vi "Actor Core.vi"(8 "error in":errorcluster, 11 "Camera_Controller in":refnum<class "Camera_Controller.lvclass">) -> (0 "error out":errorcluster, 3 "Actor out":refnum<class "Actor.lvclass">)   [LabVIEW 2023, in "Camera_Controller.lvlib" / "Camera_Controller.lvclass"]
doc: "(<B>Filename</B>: Actor Framework.lvlib:Actor.lvclass:Actor Core.vi)\n\nReceives messages to the actor, reacts to them, and initiates any error handling that may shut the actor down.\n\nDescendant classes may override this VI to append parallel tasks for the actor to complete while it handles messages. Overrides use the Call Parent Class Method node."
uses:
  Camera_Controller.lvclass
  C:/Program Files/National Instruments/LabVIEW 2023/vi.lib/ActorFramework/Actor/Actor.lvclass
  <vilib>/ActorFramework/Actor/Actor.lvclass
  <vilib>/ActorFramework/Message Enqueuer/Message Enqueuer.lvclass
  typedefs/BeamProfilerData.ctl
  typedefs/ImageProcessingParameters.ctl
  <vilib>/vision/Image Controls.llb/IMAQ Image.ctl
  typedefs/Image Type.ctl
  ConcreteClasses/ConcreteInstrumentClasses/CameraClasses/Inovance_LV/Inovance_Camera/Inovance_Camera.lvclass
  ConcreteClasses/ConcreteInstrumentClasses/CameraClasses/Hama_LV/HamaCam/Hamamatsu_Camera.lvclass
  <vilib>/ActorFramework/Actor/Actor.lvclass/Actor.ctl
  <vilib>/ActorFramework/Message Enqueuer/Message Enqueuer.lvclass/Message Enqueuer.ctl
  Camera_Controller.lvclass/Camera_Controller.ctl
  Interfaces/AbstractInstrumentClasses/Cameras_LV/CameraComm Messages/Frame Ready Msg/Frame Ready Msg.lvclass/Frame Ready Msg.ctl
  <vilib>/Utility/miscctls.llb/LVMinMaxIncTypeDef.ctl
  Interfaces/AbstractInstrumentClasses/Cameras_LV/CameraInterface Messages/GetFrame Msg/GetFrame Msg.lvclass/GetFrame Msg.ctl
  Interfaces/InitDeinitInterface/InitDeinit Messages/Init Msg/Init Msg.lvclass/Init Msg.ctl
  Interfaces/AbstractInstrumentClasses/Cameras_LV/CameraInterface Messages/StartCapture Msg/StartCapture Msg.lvclass/StartCapture Msg.ctl
  <vilib>/ActorFramework/Message Enqueuer/Message Priority.ctl
  Interfaces/AbstractInstrumentClasses/Cameras_LV/CameraInterface Messages/SingleAcquisition Msg/SingleAcquisition Msg.lvclass/SingleAcquisition Msg.ctl
  Interfaces/AbstractInstrumentClasses/Cameras_LV/CameraInterface Messages/SetExposure Msg/SetExposure Msg.lvclass/SetExposure Msg.ctl
  Interfaces/AbstractInstrumentClasses/Cameras_LV/CameraInterface Messages/Set Gain Msg/Set Gain Msg.lvclass/Set Gain Msg.ctl
  <vilib>/ActorFramework/Message Enqueuer/Init from Existing Queue.vi
  <vilib>/ActorFramework/Message Enqueuer/Enqueue.vi
  Interfaces/InitDeinitInterface/InitDeinit Messages/FindInstruments Msg/FindInstruments Msg.lvclass
  C:/Program Files/National Instruments/LabVIEW 2023/vi.lib/ActorFramework/Message/Message.lvclass
  <vilib>/ActorFramework/Stop Msg/Stop Msg.lvclass
  Interfaces/AbstractInstrumentClasses/Cameras_LV/CameraComm Messages/Frame Ready Msg/Frame Ready Msg.lvclass
  Interfaces/AbstractInstrumentClasses/Cameras_LV/CameraInterface Messages/GetFrame Msg/GetFrame Msg.lvclass
  Interfaces/InitDeinitInterface/InitDeinit Messages/DeInit Msg/DeInit Msg.lvclass
  Interfaces/InitDeinitInterface/InitDeinit Messages/Init Msg/Init Msg.lvclass
  Interfaces/AbstractInstrumentClasses/Cameras_LV/CameraInterface Messages/StartCapture Msg/StartCapture Msg.lvclass
  Interfaces/AbstractInstrumentClasses/Cameras_LV/CameraInterface Messages/StopCapture Msg/StopCapture Msg.lvclass
  Interfaces/AbstractInstrumentClasses/Cameras_LV/CameraInterface Messages/SingleAcquisition Msg/SingleAcquisition Msg.lvclass
  Interfaces/AbstractInstrumentClasses/Cameras_LV/CameraInterface Messages/SetExposure Msg/SetExposure Msg.lvclass
  Interfaces/AbstractInstrumentClasses/Cameras_LV/CameraInterface Messages/Set Gain Msg/Set Gain Msg.lvclass
  Interfaces/InitDeinitInterface/InitDeinit Messages/Disconnect Msg/Disconnect Msg.lvclass
  <vilib>/ActorFramework/Message Priority Queue/Priority Enqueue.vi
  Camera_Controller.lvlib
  typedefs/typedefs.lvlib
  <userlib>/_OpenG.lib/lvdata/lvdata.llb/openg_variant.lvlib
panel:
  out "Cam Enqueuer Init":bool
  out "Stopping":bool=TRUE
  out "error out Instr":errorcluster
  out "Instrument Address":string[](array[string])
  out "Orca Enqueuer":refnum<class "Message Enqueuer.lvclass">
  out "Self Enqueuer":refnum<class "Message Enqueuer.lvclass">
  out "Inovance Enqueuer":refnum<class "Message Enqueuer.lvclass">
  out "Address Var":variant
  out "Error Var":variant
  in  "Beam Profiler Kwargs":cluster{"Pixel Size":dbl}={"Pixel Size"=2.5}
  in  "Beam Profiler Data":T1
  out "Camera Enqueuer":refnum<class "Message Enqueuer.lvclass">
  out "Brand":string[](array[string])
  out "Custom ROI":i32[](array[numeric])
  in  "Tab Control":enum32{"Camera", "Options"}(tab)
  in  "Beam Profile":bool
  in  "File Path":path
  in  "File Name":string
  in  "Save":bool
  out "Image Processed":T2(plugin-control) caption="Image"
  in  "HROI Pos":u16
  in  "HROI":bool
  out "VI":refnum<vi>
  out "Image":T2(plugin-control)
  out "Capturing":bool=TRUE
  out "FPS":dbl
  in  "Camera":u16(ring)
  out "Initialized":bool=TRUE
  in  "Open Camera":bool
  in  "Gain":dbl=1.0 min=1.0 max=32.0 step=0.1
  in  "Exposure":dbl=0.01 min=0.01 max=10000.0 step=0.01
  in  "Acquire":bool
  in  "Live":bool
  out "ROI Graph":cluster{"x0":sgl, "dx":sgl, "Pixels Line":sgl[]}(graph)={"x0"=0.0, "dx"=1.0, "Pixels Line"=[1.0, 0.0, 0.0, 0.0, 0.0, 0.0, 0.0, 0.0, 0.0, 0.0, 0.0, 0.0, 0.0, 0.0, 0.0, 0.0, 0.0, 0.0, 0.0, 0.0, 0.0, 0.0, 0.0, 0.0, 0.0, 0.0, 0.0, 0.0, 0.0, 0.0, 0.0, 0.0, 0.0, 0.0, 0.0, 0.0, 0.0, 0.0, 0.0, 0.0, 0.0, 0.0, 0.0, 0.0, 0.0, 0.0, 0.0, 0.0, 0.0, 0.0, 0.0, 0.0, 0.0, 0.0, 0.0, 0.0, 0.0, 0.0, 0.0, 0.0, 0.0, 0.0, 0.0, 0.0, 0.0, 0.0, 0.0, 0.0, 0.0, 0.0, 0.0, 0.0, 0.0, 0.0, 0.0, 0.0, 0.0, 0.0, 0.0, 0.0, 0.0, 0.0, 0.0, 0.0, 0.0, 0.0, 0.0, 0.0, 0.0, 0.0, 0.0, 0.0, 0.0, 0.0, 0.0, 0.0, 0.0, 0.0, 0.0, 0.0, 0.0, 0.0, 0.0, 0.0, 0.0, 0.0, 0.0, 0.0, 0.0, 0.0, 0.0, 0.0, 0.0, 0.0, 0.0, 0.0, 0.0, 0.0, 0.0, 0.0, 0.0, 0.0, 0.0, 0.0, 0.0, 0.0, 0.0, 0.0, 0.0, 0.0, 0.0, 0.0, 0.0, 0.0, 0.0, 0.0, 0.0, 0.0, 0.0, 0.0, 0.0, 0.0, 0.0, 0.0, 0.0, 0.0, 0.0, 0.0, 0.0, 0.0, 0.0, 0.0, 0.0, 0.0, 0.0, 0.0, 0.0, 0.0, 0.0, 0.0, 0.0, 0.0, 0.0, 0.0, 0.0, 0.0, 0.0, 0.0, 0.0, 0.0, 0.0, 0.0, 0.0, 0.0, 0.0, 0.0, 0.0, 0.0, 0.0, 0.0, 0.0, 0.0, 0.0, 0.0, 0.0, 0.0, 0.0, 0.0, 0.0, 0.0, 0.0, 0.0, 0.0, 0.0, 0.0, 0.0, 0.0, 0.0, 0.0, 0.0, 0.0, 0.0, 0.0, 0.0, 0.0, 0.0, 0.0, 0.0, 0.0, 0.0, 0.0, 0.0, 0.0, 0.0, 0.0, 0.0, 0.0, 0.0, 0.0, 0.0, 0.0, 0.0, 0.0, 0.0, 0.0, 0.0, 0.0, 0.0, 0.0, 0.0, 0.0, 0.0, 0.0, 0.0, 0.0, 0.0, 0.0, 0.0, 0.0, 0.0, 0.0, 0.0, 0.0, 0.0, 0.0, 0.0, 0.0, 0.0, 0.0, 0.0, 0.0, 0.0, 0.0, 0.0, 0.0, 0.0]}
  in  "Mode":enum16{"ROI", "Image"}(ring)
  out "ROI Parameters":cluster{"Count":sgl, "Size(um)":sgl} {"Size(um)" min=0 max=255 step=0.1 format="%.2f"; "Count" min=0 max=255 step=0.1 format="%.2f"}
  in  "Refresh Button":bool
  in  "Stop":bool
  in  "Auto?":bool
  in  "Log?":bool
  in  "Manual":cluster{sgl, sgl}(slide)={100.0, 255.0} caption="Threshold Range" scale=0.0..65535.0
  out "Beam Profile":T1
  out "Image Preview":T2(plugin-control) caption="Image"
  out "Calibration Axes":u8[][](graph)
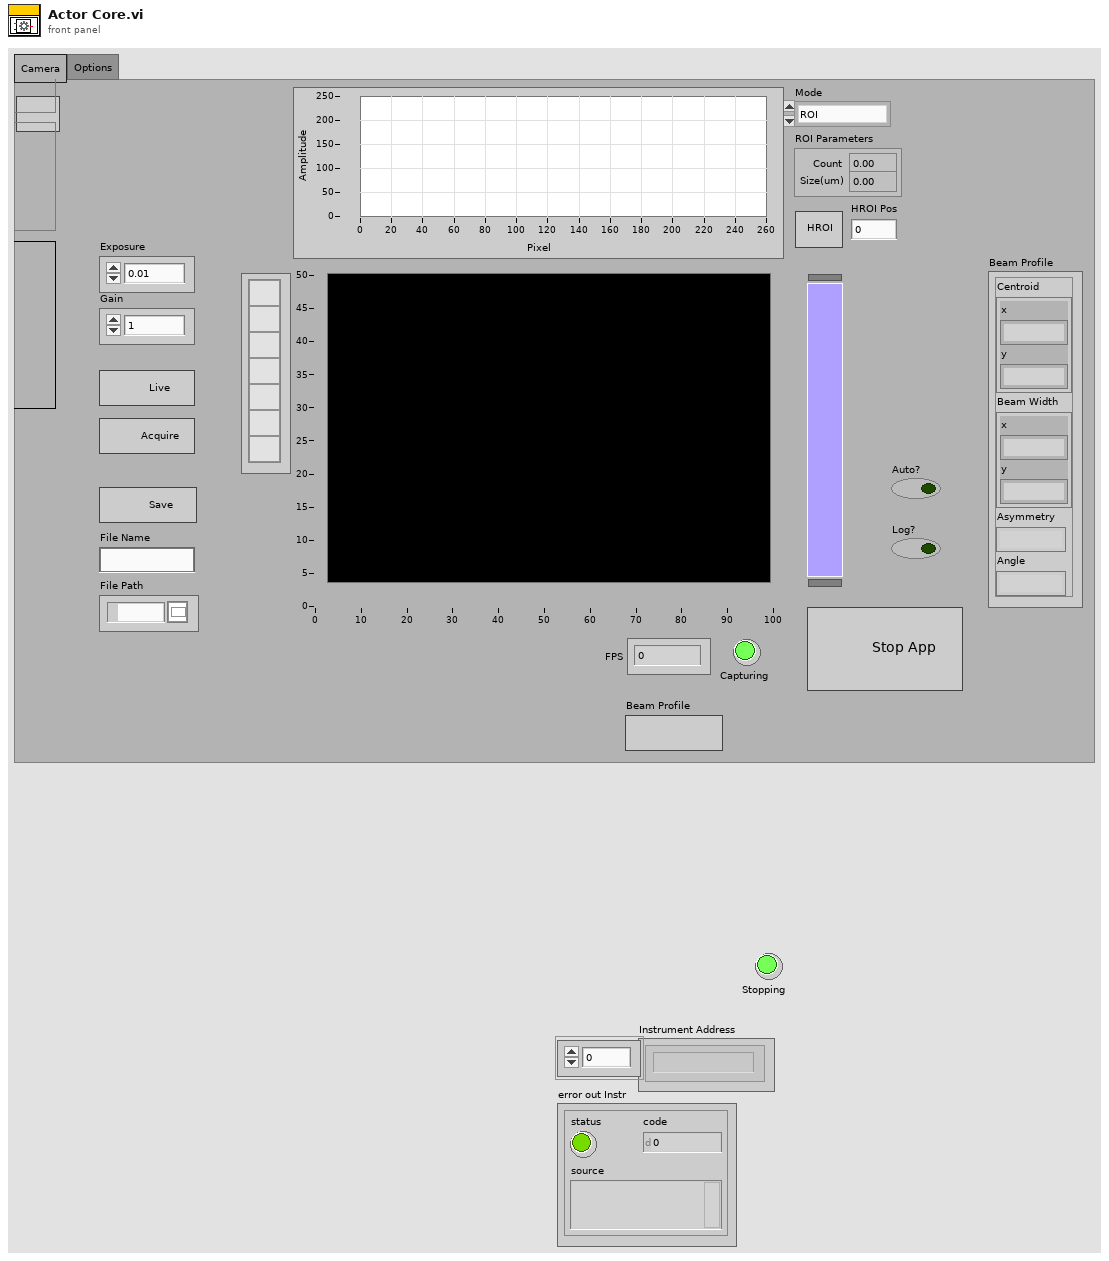
[diagram p1: front panel]
types:
  T1 = typedef "BeamProfilerData.ctl" = cluster{"Centroid":cluster{"x":string, "y":string}, "Beam Width":cluster{"x":string, "y":string}, "Asymmetry":string, "Angle":string}
  T2 = typedef "IMAQ Image.ctl" = refnum<image>
  T3 = typedef "typedefs.lvlib/ImageProcessingParameters.ctl" = cluster{"Mode":enum16{"ROI", "Image"}, "Manual LUT":cluster{"Minimum":dbl, "Maximum":dbl}, "ImageProcessed":T2, "Image ":T2, "Log?":bool, "Auto?":bool, "ROI":cluster{"Global Rectangle":i32[], "Contours":cluster{"Contour Type":u32, "ROI Type":u32, "Points":i32[]}[]}, "ROI Parameters":cluster{"Count":sgl, "Size(um)":sgl}, "Image X":i32, "Image Y":i32, "Horizontal ROI":cluster{"Global Rectangle":i32[], "Contours":cluster{"Contour Type":u32, "ROI Type":u32, "Points":i32[]}[]}, "HROI Pos":u16, "Custom ROI":cluster{"Global Rectangle":i32[], "Contours":cluster{"Contour Type":u32, "ROI Type":u32, "Points":i32[]}[]}, "Intensity Graph":u8[][], "Image Type":T4, "ImagePreview":T2}
  T4 = typedef "typedefs.lvlib/Image Type.ctl" = u32
  T5 = enum8{"Enabled", "Disabled", "Disabled and Grayed Out"}
  T6 = typedef "LVMinMaxIncTypeDef.ctl" = cluster{"Maximum":dbl, "Minimum":dbl, "Increment":dbl}
  T7 = cluster{"Global Rectangle":i32[], "Contours":cluster{"Contour Type":u32, "ROI Type":u32, "Points":i32[]}[]}
  T8 = typedef "Image Type" = u32
  T9 = typedef "Actor Framework.lvlib/Message Enqueuer.lvclass/Message Priority.ctl" = enum16{"Low", "Normal", "High"}
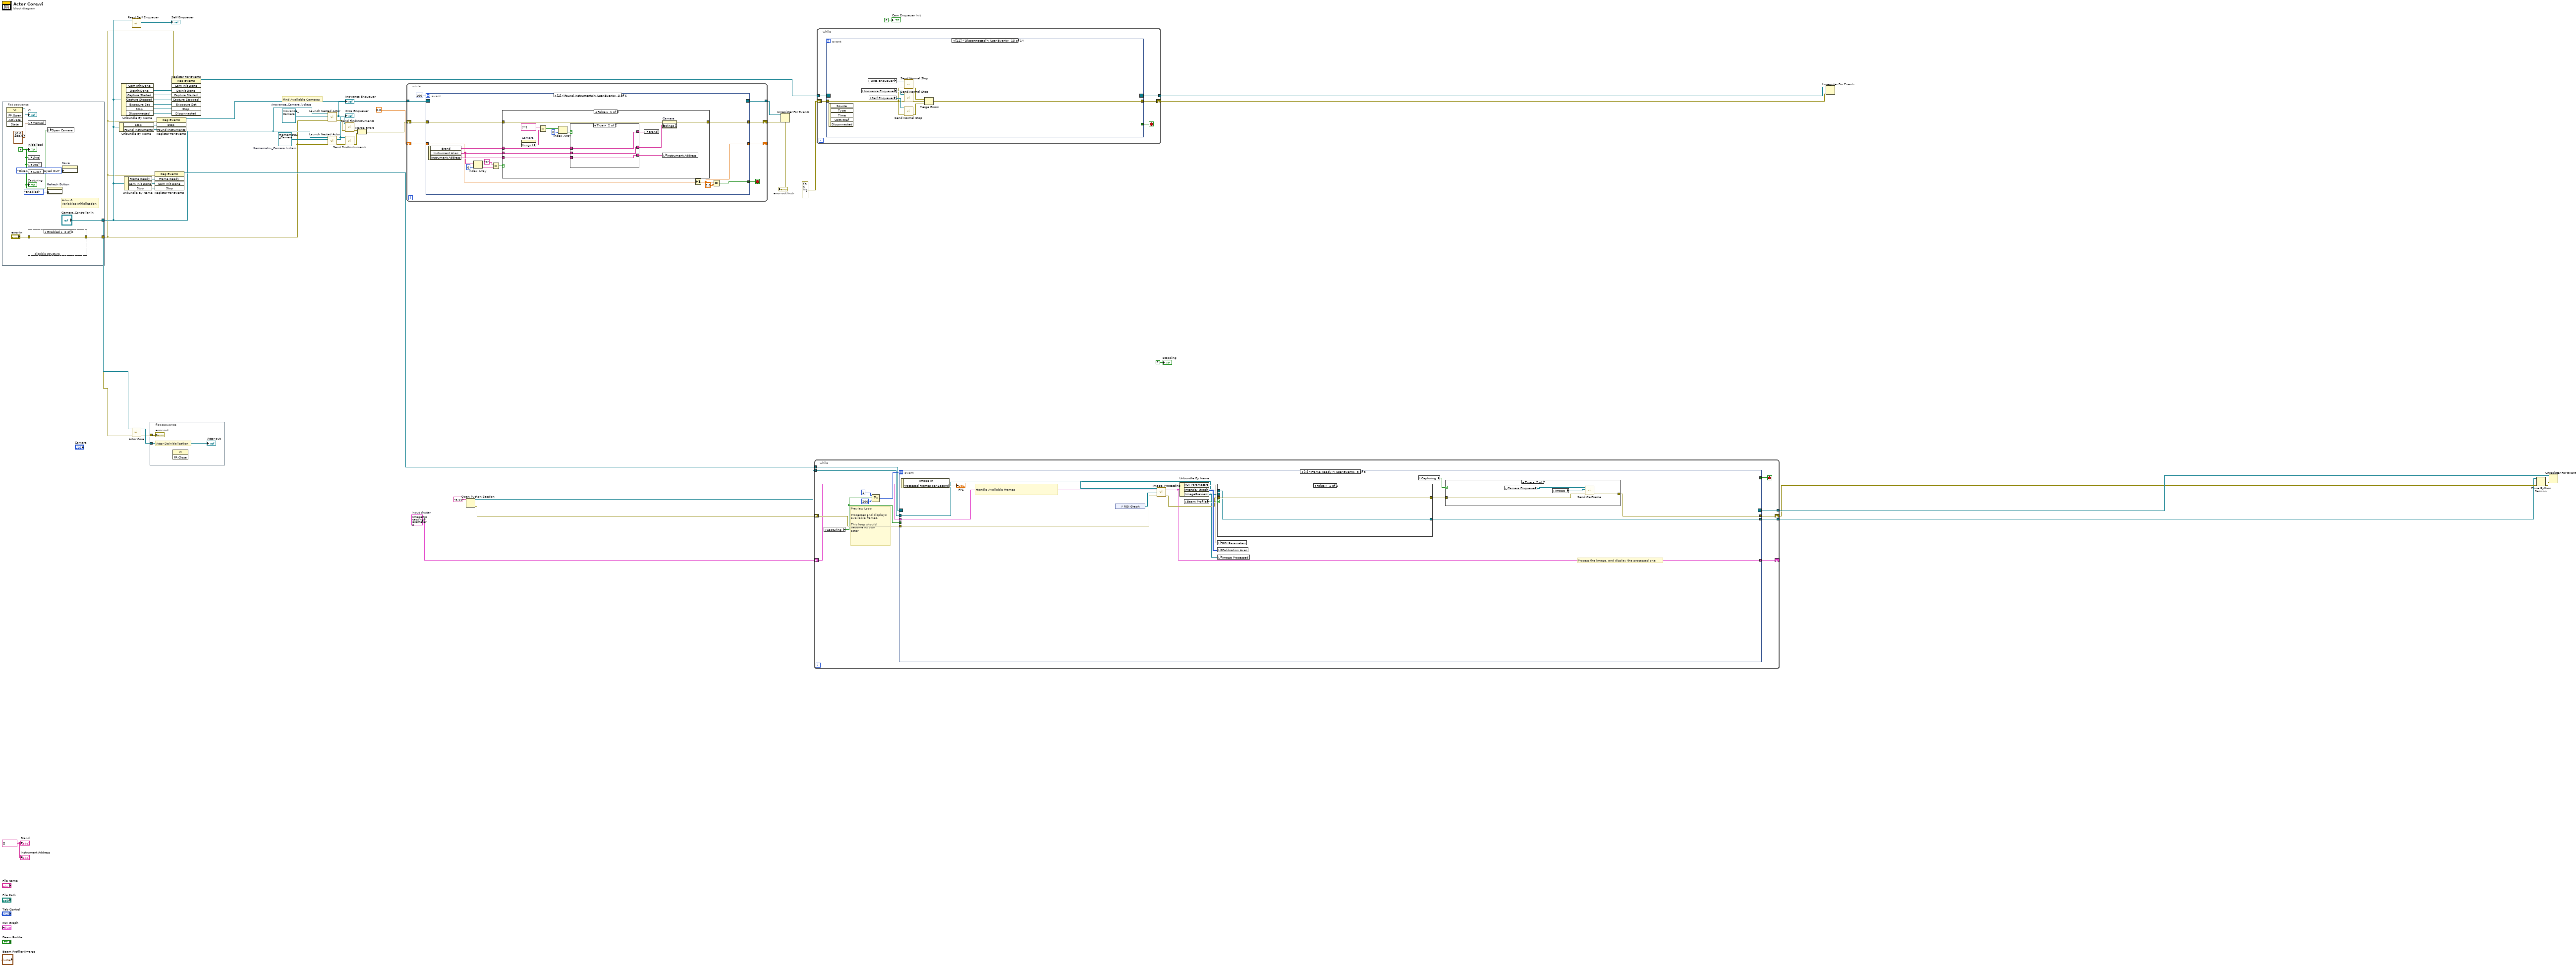
[diagram p0: block diagram]
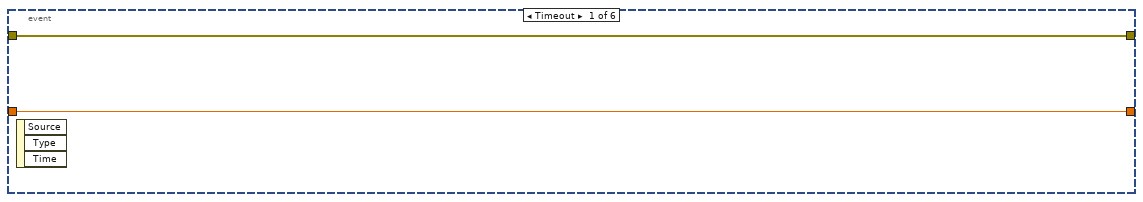
[diagram p2: hidden frame]
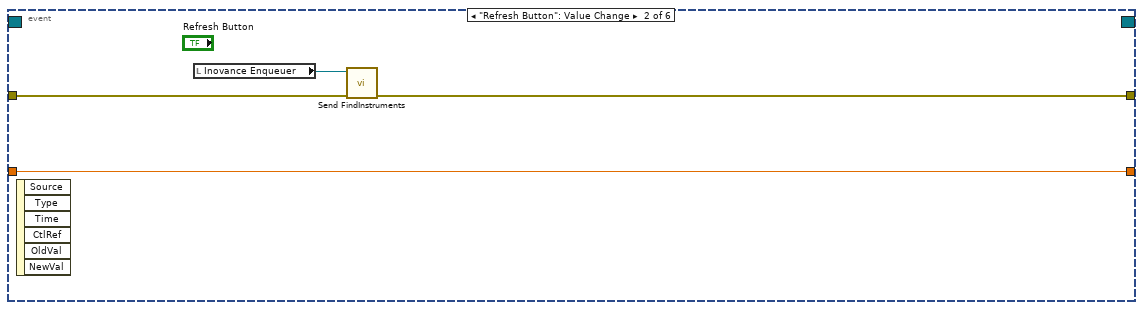
[diagram p3: hidden frame]
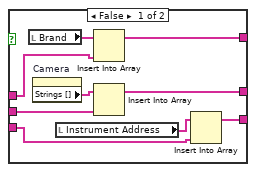
[diagram p4: hidden frame]
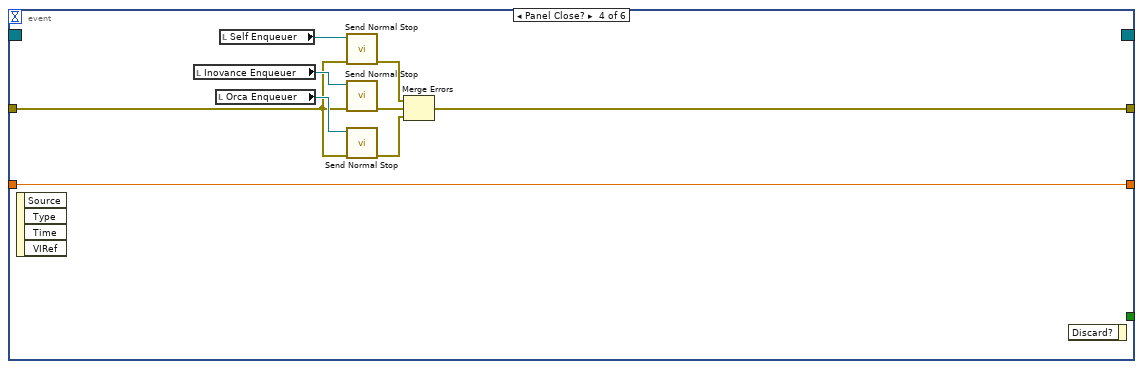
[diagram p6: hidden frame]
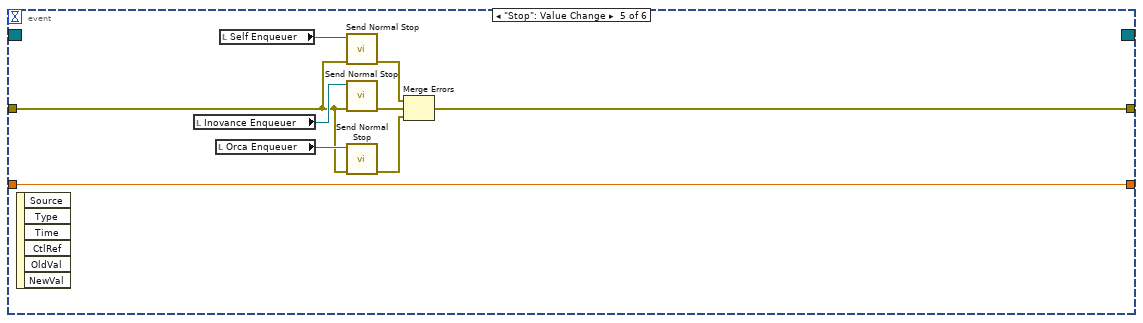
[diagram p7: hidden frame]
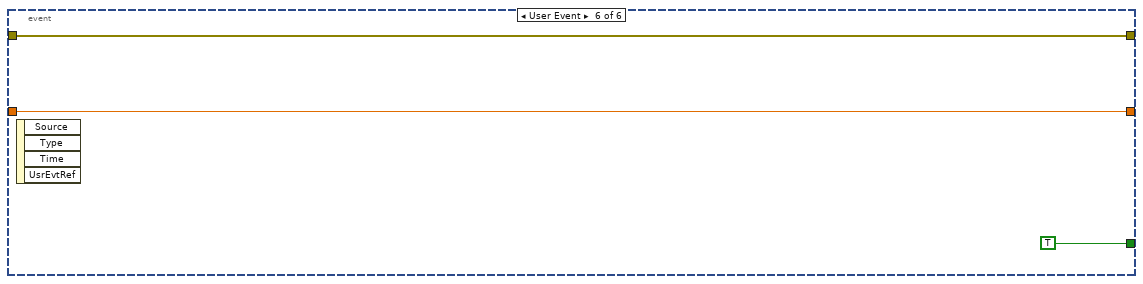
[diagram p8: hidden frame]
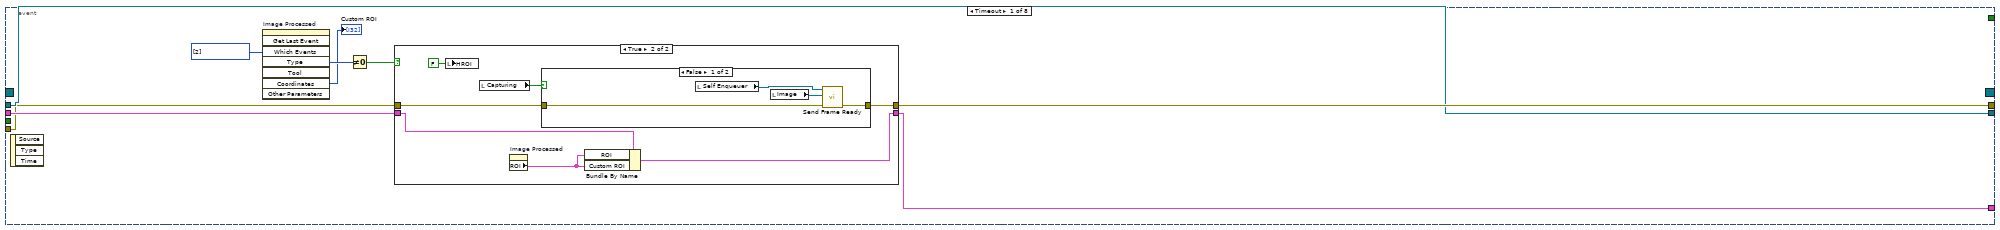
[diagram p9: hidden frame]
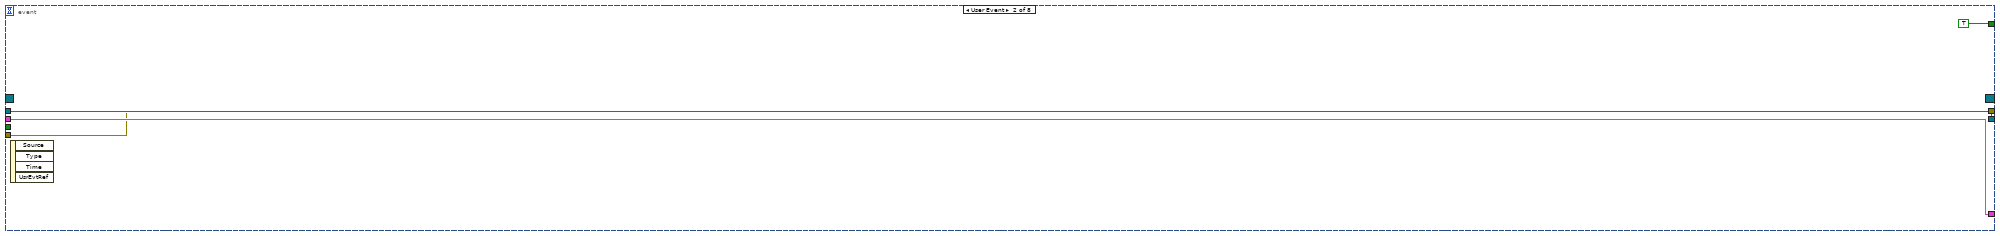
[diagram p12: hidden frame]
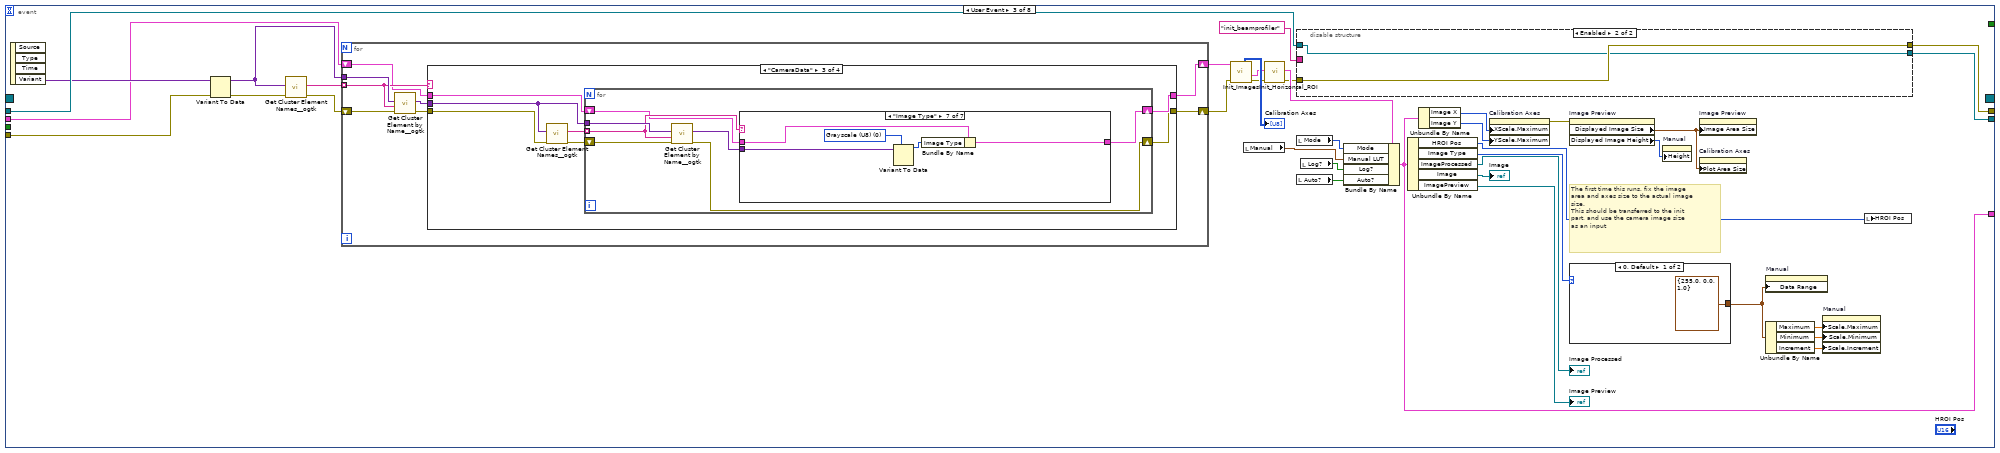
[diagram p13: hidden frame]
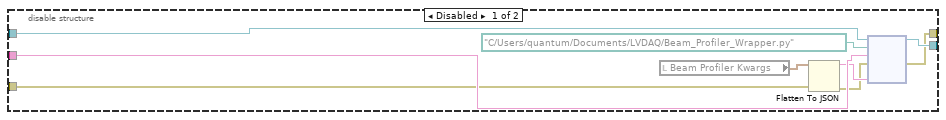
[diagram p14: hidden frame]
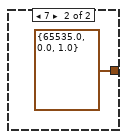
[diagram p15: hidden frame]
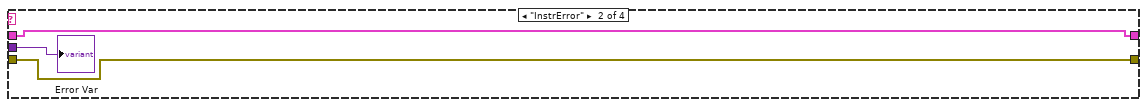
[diagram p17: hidden frame]
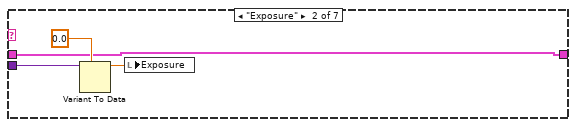
[diagram p19: hidden frame]
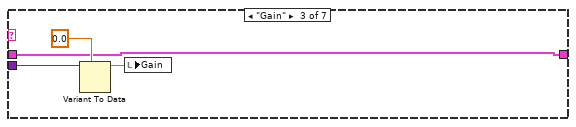
[diagram p20: hidden frame]
diagram:
  w13 = refnum<class "Hamamatsu_Camera.lvclass"> refnum  # Hamamatsu_Camera.lvclass
  w14 = refnum<class "Inovance_Camera.lvclass"> refnum  # :Inovance_Camera.lvclass
  w19 = string[] [] ("Brand")
  w37 = T3 {"Mode"=enum."Image", "Manual LUT"={"Minimum"=0.0, "Maximum"=0.0}, "ImageProcessed"=refnum, "Image "=refnum, "Log?"=FALSE, "Auto?"=FALSE, "ROI"={"Global Rectangle"=[], "Contours"=[]}, "ROI Parameters"={"Count"=0.0, "Size(um)"=0.0}, "Image X"=0, "Image Y"=0, "Horizontal ROI"={"Global Rectangle"=[], "Contours"=[]}, "HROI Pos"=0, "Custom ROI"={"Global Rectangle"=[], "Contours"=[]}, "Intensity Graph"=[], "Image Type"=7, "ImagePreview"=refnum}  # input cluster
  # "Find Available Cameras"
  n1 = flat-sequence {
    tunnel: ["Camera_Controller in"] -> w22
    tunnel: [w49] -> w2
    frame #0 {
      w53 = FALSE ("Capturing")
      # "Actor & \nVariables Initialization"
      n2 = invoke class="VI" method="FP.Open"() -> (reference out=→"VI":refnum<vi>)  [unwired: 5 in, 4 out]
      n3 = local write "Manual"(cluster{sgl, sgl} {0.0, 255.0} ("Manual")) -> ()
      n4 = local write "Live"(w53) -> ()
      n5 = local write "Log?"(w53) -> ()
      n6 = local write "Auto?"(w53) -> ()
      n7 = disable-structure shown="Enabled" {
        disable-tunnel: "error in" -> [w57 w61]
        disable-tunnel: [w56 w61] -> w49
        frame Disabled {
          n8 = Initialize Array("" ("element"), 0 ("dimension size")) -> (w60:string[])
          n9 = property on="Camera" class="Ring (strict)"(error in=w57, "Strings []"=w60) -> (error out=w56:errorcluster)  [unwired: 1 in, 1 out]
        }
        frame Enabled {
        }
      }
      n10 = local write "Open Camera"(w53) -> ()
      n11 = property on="Refresh Button" class="Bool"("DisabledEnum"=T5."Enabled" ("Disabled")) -> ()  [unwired: 2 in, 2 out]
      n12 = property on="Save" class="Bool"("DisabledEnum"=T5."Disabled and Grayed Out" ("Disabled")) -> ()  [unwired: 2 in, 2 out]
      "Capturing" <- w53
      "Initialized" <- w53
    }
  }
  n13 = Unbundle By Name(w22) -> ("Stop"=w35:refnum<user-event>, "Found Instruments"=w27:refnum<user-event>)
  n14 = Unbundle By Name(w22) -> ("Cam Init Done"=w23:refnum<user-event>, "DeInit Done"=w44:refnum<user-event>, "Capture Started"=w43:refnum<user-event>, "Capture Stopped"=w42:refnum<user-event>, "Exposure Set"=w41:refnum<user-event>, "Stop"=w36:refnum<user-event>, "Disconnected"=w4:refnum<user-event>)
  n15 = Unbundle By Name(w22) -> ("Frame Ready"=w25:refnum<user-event>, "Cam Init Done"=w24:refnum<user-event>, "Stop"=w8:refnum<user-event>)
  n16 = call <vilib>:"Read Self Enqueuer.vi"("Actor"=w22) -> ("Self Enqueuer"=→"Self Enqueuer":refnum<class "Message Enqueuer.lvclass">)  [unwired: 10 in]
  n17 = call-parent "Actor Core.vi"("error in"=w2, "Actor in"=w22) -> ("error out"=w46:errorcluster, "Actor out"=w47:refnum<class "Actor.lvclass">)  [unwired: 8 in]
  n18 = flat-sequence {
    tunnel: w47 -> [w63]
    tunnel: w46 -> [w62]
    frame #0 {
      # "Actor Deinitialization"
      n19 = invoke class="VI" method="FP.Close"() -> ()  [unwired: 3 in, 3 out]
      "error out" <- w62
      "Actor out" <- w63
    }
  }
  n20 = register-events(error in=w2, w25, w24, w8) -> (reference out=w34:refnum<event-registration>)  [unwired: 1 in, 1 out]
  n21 = register-events(error in=w2, w35, w27) -> (reference out=w5:refnum<event-registration>)  [unwired: 1 in, 1 out]
  n22 = register-events(error in=w2, w23, w44, w43, w42, w41, w36, w4) -> (reference out=w45:refnum<event-registration>)  [unwired: 1 in, 1 out]
  n23 = call <vilib>:"Launch Nested Actor.vi"("error in (no error)"=w2, "Nested Actor"=w14, "Caller Actor in"=w22) -> ("error out"=w16:errorcluster, "Nested Actor's Enqueuer"=w15:refnum<class "Message Enqueuer.lvclass">)  [unwired: 6 in, 1 out]
  "Inovance Enqueuer" <- w15
  n24 = call <vilib>:"Launch Nested Actor.vi"("error in (no error)"=w2, "Nested Actor"=w13, "Caller Actor in"=w22) -> ("error out"=w9:errorcluster, "Nested Actor's Enqueuer"=w12:refnum<class "Message Enqueuer.lvclass">)  [unwired: 6 in, 1 out]
  "Orca Enqueuer" <- w12
  n25 = call "Send FindInstruments.vi"("error in (no error)"=w16, "Message Enqueuer"=w15) -> ("error out"=w10:errorcluster)  [unwired: 8 in, 1 out]
  n26 = call "Send FindInstruments.vi"("error in (no error)"=w9, "Message Enqueuer"=w12) -> ("error out"=w11:errorcluster)  [unwired: 8 in, 1 out]
  n27 = Merge Errors(w10, w11) -> (w21:errorcluster)
  n28 = while {
    shift-right: [w71] -> w17
    shift-left: w21 -> [w70]
    tunnel: w5 -> [w68]
    shift-right: [w65] -> _
    shift-left: 0.0 -> [w66]
    tunnel: [w64] -> w18
    stop <- w69 stop-if-true
    n29 = event shown="[2] <Found Instruments>: User Event" {
      selector: w68 -> [_ _ _ _ _ _]
      dyn-events: [_ _ _ _ _ _] -> w64
      timeout: 100 -> [_ _ _ _ _ _]
      tunnel: [_ _ w89 _ _ TRUE] -> w69
      tunnel: [w73 w76 w82 w121 w130 w136] -> w71
      tunnel: w70 -> [w73 w77 w83 w118 w126 w136]
      tunnel: w66 -> [w72 w74 w79 w120 w129 w135]
      tunnel: [w72 w74 w78 w120 w129 w135] -> w65
      event Timeout {
        n30 = event-data() -> ()  [unwired: 1 in, 3 out]
      }
      event "Refresh Button": Value Change {
        n31 = event-data() -> ()  [unwired: 1 in, 6 out]
        n32 = local read "Inovance Enqueuer"() -> (w75:refnum<class "Message Enqueuer.lvclass">)
        n33 = call "Send FindInstruments.vi"("error in (no error)"=w77, "Message Enqueuer"=w75) -> ("error out"=w76:errorcluster)  [unwired: 8 in, 1 out]
      }
      event User Event {
        n34 = event-data() -> ("Brand"=w87:string[], "Instrument Alias"=w80:string[], "Instrument Address"=w81:string[])  [unwired: 1 in]
        n35 = Index Array(array=w80, index=0) -> (element=w85:string)
        n36 = Equal?(x="0", y=w85) -> (x = y?=w86:bool)
        n37 = case shown="False" w86 {
          tunnel: w80 -> [w103 _]
          tunnel: w81 -> [w102 _]
          tunnel: w87 -> [w101 _]
          tunnel: w83 -> [w98 w116]
          tunnel: [w96 w116] -> w82
          frame False {
            n38 = property on="Camera" class="Ring (strict)"() -> ("Strings []"=w93:string[])  [unwired: 2 in, 2 out]
            n39 = Equal?(x=string[] [""] ("Strings []"), y=w93) -> (x = y?=w91:bool[])
            n40 = Index Array(array=w91, index=0) -> (element=w94:bool)
            n41 = case shown="True" w94 {
              tunnel: w103 -> [w111 w115]
              tunnel: [w110 w115] -> w97
              tunnel: w101 -> [w109 w113]
              tunnel: [w106 w114] -> w99
              tunnel: [w105 w113] -> w100
              tunnel: w102 -> [w104 w114]
              frame False {
                n42 = local read "Brand"() -> (w107:string[])
                n43 = property on="Camera" class="Ring (strict)"() -> ("Strings []"=w112:string[])  [unwired: 2 in, 2 out]
                n44 = local read "Instrument Address"() -> (w108:string[])
                n45 = Insert Into Array(array=w107, new element=w109) -> (w105:string[])  [unwired: 1 in]
                n46 = Insert Into Array(array=w112, new element=w111) -> (w110:string[])  [unwired: 1 in]
                n47 = Insert Into Array(array=w108, new element=w104) -> (w106:string[])  [unwired: 1 in]
              }
              frame True {
              }
            }
            n48 = local write "Brand"(w100) -> ()
            n49 = property on="Camera" class="Ring (strict)"(error in=w98, "Strings []"=w97) -> (error out=w96:errorcluster)  [unwired: 1 in, 1 out]
            n50 = local write "Instrument Address"(w99) -> ()
          }
          frame True {
          }
        }
        n51 = Increment(x=w79) -> (x+1=w78:dbl)
        n52 = Equal?(x=w78, y=2.0) -> (x = y?=w89:bool)
      }
      event Panel Close? {
        n53 = event-data() -> ()  [unwired: 1 in, 4 out]
        n54 = local read "Inovance Enqueuer"() -> (w124:refnum<class "Message Enqueuer.lvclass">)
        n55 = local read "Orca Enqueuer"() -> (w119:refnum<class "Message Enqueuer.lvclass">)
        n56 = local read "Self Enqueuer"() -> (w125:refnum<class "Message Enqueuer.lvclass">)
        n57 = call <vilib>:"Send Normal Stop.vi"("error in (no error)"=w118, "Message Enqueuer"=w125) -> ("error out"=w123:errorcluster)  [unwired: 9 in]
        n58 = call <vilib>:"Send Normal Stop.vi"("error in (no error)"=w118, "Message Enqueuer"=w124) -> ("error out"=w122:errorcluster)  [unwired: 9 in]
        n59 = call <vilib>:"Send Normal Stop.vi"("error in (no error)"=w118, "Message Enqueuer"=w119) -> ("error out"=w117:errorcluster)  [unwired: 9 in]
        n60 = Merge Errors(w123, w122, w117) -> (w121:errorcluster)
        n61 = event-data() -> ()  [unwired: 2 in, 1 out]
      }
      event "Stop": Value Change {
        n62 = event-data() -> ()  [unwired: 1 in, 6 out]
        n63 = local read "Inovance Enqueuer"() -> (w133:refnum<class "Message Enqueuer.lvclass">)
        n64 = local read "Orca Enqueuer"() -> (w128:refnum<class "Message Enqueuer.lvclass">)
        n65 = local read "Self Enqueuer"() -> (w134:refnum<class "Message Enqueuer.lvclass">)
        n66 = call <vilib>:"Send Normal Stop.vi"("error in (no error)"=w126, "Message Enqueuer"=w134) -> ("error out"=w132:errorcluster)  [unwired: 9 in]
        n67 = call <vilib>:"Send Normal Stop.vi"("error in (no error)"=w126, "Message Enqueuer"=w133) -> ("error out"=w131:errorcluster)  [unwired: 9 in]
        n68 = call <vilib>:"Send Normal Stop.vi"("error in (no error)"=w126, "Message Enqueuer"=w128) -> ("error out"=w127:errorcluster)  [unwired: 9 in]
        n69 = Merge Errors(w132, w131, w127) -> (w130:errorcluster)
      }
      event User Event {
        n70 = event-data() -> ()  [unwired: 1 in, 4 out]
      }
    }
  }
  n71 = Open Python Session(python version="3.11" ("Python version")) -> (session out=w33:refnum<k35>, error out=w31:errorcluster)  [unwired: 2 in]
  n72 = Unregister For Events(event registration refnum=w18, error in=w17) -> (error out=→"error out Instr":errorcluster)
  n73 = while {
    tunnel: w34 -> [w150]
    tunnel: [w149] -> w40
    shift-right: [w139] -> w30
    shift-left: w31 -> [w148]
    shift-right: [w140] -> _
    shift-left: w37 -> [w143]
    tunnel: w33 -> [w142]
    tunnel: [w141] -> w28
    stop <- w138 stop-if-true
    # "Preview Loop\n\nProcesses and displays\navailable frames.\n\nThis loop should\nbecome its own\nactor"
    n74 = local read "Capturing"() -> (w144:bool)
    n75 = Select(t=1, s=w144, f=200) -> (s? t:f=w145:i32)
    n76 = event shown="[4] <Frame Ready>: User Event" {
      selector: w150 -> [_ _ _ _ _ _ _ _]
      dyn-events: [_ _ _ _ _ _ _ _] -> w149
      timeout: w145 -> [_ _ _ _ _ _ _ _]
      tunnel: [w155 w174 w212 w290 w296 w336 w360 w370] -> w139
      tunnel: w148 -> [w151 w174 w209 w292 w309 w337 w361 w371]
      tunnel: w144 -> [_ _ _ _ _ _ _ _]
      tunnel: w143 -> [w157 w176 w206 w288 w306 w338 w359 w373]
      tunnel: [w152 w176 w188 w288 w298 w331 w354 w368] -> w140
      tunnel: w142 -> [w153 w177 w214 w289 w301 w332 w355 w369]
      tunnel: [w153 w177 w213 w289 w300 w332 w355 w369] -> w141
      tunnel: [_ TRUE _ _ _ _ _ _] -> w138
      event Timeout {
        w158 = i32[] [2] items=["No Event"=0, "Click Event"=1, "Draw Event"=2, "Size Event"=4, "Scroll Event"=5, "Double Click Event"=8] ("Which Events")
        n77 = event-data() -> ()  [unwired: 1 in, 3 out]
        n78 = invoke on="Image Processed" class="ImageControl" method="Get Last Event"("Which Events"=w158) -> ("Type"=w159:i32, "Coordinates"=→"Custom ROI":i32[])  [unwired: 7 in, 6 out]
        n79 = Not Equal To 0?(x=w159) -> (x != 0?=w156:bool)
        n80 = case shown="True" w156 {
          tunnel: w157 -> [w161 w168]
          tunnel: [w161 w167] -> w152
          tunnel: w151 -> [w160 w165]
          tunnel: [w160 w164] -> w155
          frame False {
          }
          frame True {
            n81 = local write "HROI"(FALSE ("HROI")) -> ()
            n82 = local read "Capturing"() -> (w166:bool)
            n83 = property on="Image Processed" class="ImageControl"() -> ("ROI"=w163:T7)  [unwired: 2 in, 2 out]
            n84 = case shown="False" w166 {
              tunnel: w165 -> [w172 w173]
              tunnel: [w171 w173] -> w164
              frame False {
                n85 = local read "Self Enqueuer"() -> (w169:refnum<class "Message Enqueuer.lvclass">)
                n86 = local read "Image"() -> (w170:T2)
                n87 = call "Send Frame Ready.vi"("error in (no error)"=w172, "Image In"=w170, "Message Enqueuer"=w169) -> ("error out"=w171:errorcluster)  [unwired: 7 in, 1 out]
              }
              frame True {
              }
            }
            n88 = Bundle By Name(cluster=w168, "ROI"=w163, "Custom ROI"=w163) -> (w167:T3)
          }
        }
      }
      event User Event {
        n89 = event-data() -> ()  [unwired: 1 in, 4 out]
      }
      event User Event {
        # "The first time this runs, fix the image\narea and axes size to the actual image\nsize.\nThis should be transferred to the init\npart, and use the camera image size\nas an input"
        n90 = event-data() -> ("Variant"=w210:variant)  [unwired: 1 in, 3 out]
        n91 = Variant To Data(error in=w209, Variant=w210) -> (data=w207:variant, error out=w195:errorcluster)  [unwired: 1 in]
        n92 = call <userlib>:"Get Cluster Element Names__ogtk.vi"("error in (no error)"=w195, "Cluster"=w207) -> ("error out"=w196:errorcluster, "Element Names"=w208:string[])  [unwired: 8 in]
        n93 = for {
          tunnel: w208 -> [w234] mode=indexing
          tunnel: w207 -> [w235]
          shift-right: [w229] -> w194
          shift-left: w196 -> [w230]
          shift-right: [w228] -> w205
          shift-left: w206 -> [w232]
          n94 = call <userlib>:"Get Cluster Element by Name__ogtk.vi"("error in (no error)"=w230, "Element Name"=w234, "Cluster"=w235) -> ("error out"=w231:errorcluster, "VElement"=w233:variant)  [unwired: 6 in, 1 out]
          n95 = case shown="\"CameraData\"" w234 {
            tunnel: w233 -> [_ w240 w246 w287]
            tunnel: w232 -> [w237 w239 w245 w286]
            tunnel: [w237 w239 w244 w286] -> w228
            tunnel: w231 -> [w236 w238 w243 w285]
            tunnel: [w236 w238 w241 w285] -> w229
            frame "False", Default {
            }
            frame "InstrError" {
              "Error Var" <- w240
            }
            frame "CameraData" {
              n96 = call <userlib>:"Get Cluster Element Names__ogtk.vi"("error in (no error)"=w243, "Cluster"=w246) -> ("error out"=w242:errorcluster, "Element Names"=w247:string[])  [unwired: 8 in]
              n97 = for {
                tunnel: w247 -> [w253] mode=indexing
                tunnel: w246 -> [w254]
                shift-right: [w248] -> w241
                shift-left: w242 -> [w249]
                shift-right: [w250] -> w244
                shift-left: w245 -> [w251]
                n98 = call <userlib>:"Get Cluster Element by Name__ogtk.vi"("error in (no error)"=w249, "Element Name"=w253, "Cluster"=w254) -> ("error out"=w248:errorcluster, "VElement"=w252:variant)  [unwired: 6 in, 1 out]
                n99 = case shown="\"Image Type\"" w253 {
                  tunnel: w252 -> [_ w259 w263 w268 w273 w279 w284]
                  tunnel: w251 -> [w255 w256 w260 w266 w270 w274 w283]
                  tunnel: [w255 w256 w260 w265 w269 w274 w282] -> w250
                  frame "False", Default {
                  }
                  frame "Exposure" {
                    n100 = Variant To Data(type=0.0, Variant=w259) -> (data=w257:dbl)  [unwired: 1 in, 1 out]
                    n101 = local write "Exposure"(w257) -> ()
                  }
                  frame "Gain" {
                    n102 = Variant To Data(type=0.0, Variant=w263) -> (data=w261:dbl)  [unwired: 1 in, 1 out]
                    n103 = local write "Gain"(w261) -> ()
                  }
                  frame "Image XDim" {
                    n104 = Variant To Data(type=u16 0 ("Image XDim"), Variant=w268) -> (data=w264:u16)  [unwired: 1 in, 1 out]
                    n105 = Bundle By Name(cluster=w266, "Image X"=w264) -> (w265:T3)
                  }
                  frame "Image YDim" {
                    n106 = Variant To Data(type=u16 0 ("Image XDim"), Variant=w273) -> (data=w271:u16)  [unwired: 1 in, 1 out]
                    n107 = Bundle By Name(cluster=w270, "Image Y"=w271) -> (w269:T3)
                  }
                  frame "Pixel Size" {
                    n108 = Variant To Data(type=0.0 ("Image XDim"), Variant=w279) -> (data=w275:dbl)  [unwired: 1 in, 1 out]
                    n109 = local read "Beam Profiler Kwargs"() -> (w276:cluster{"Pixel Size":dbl})
                    n110 = Bundle By Name(cluster=w276, "Pixel Size"=w275) -> (w277:cluster{"Pixel Size":dbl})
                    n111 = local write "Beam Profiler Kwargs"(w277) -> ()
                  }
                  frame "Image Type" {
                    w280 = T8 0 items=["Grayscale (U8)", "Grayscale (I16)", "Grayscale (SGL)", "Complex (CSG)", "RGB (U32)", "HSL (U32)", "RGB (U64)", "Grayscale (U16)"] ("Image Type")
                    n112 = Variant To Data(type=w280, Variant=w284) -> (data=w281:T8)  [unwired: 1 in, 1 out]
                    n113 = Bundle By Name(cluster=w283, "Image Type"=w281) -> (w282:T3)
                  }
                }
              }
            }
            frame "Address" {
              "Address Var" <- w287
            }
          }
        }
        n114 = call "Init_Images.vi"("error in (no error)"=w194, "input cluster in"=w205) -> ("error out"=w193:errorcluster, "input cluster out"=w197:T3, "Image Pixels (U8)"=→"Calibration Axes":u8[][])  [unwired: 7 in]
        n115 = local read "Manual"() -> (w203:cluster{sgl, sgl})
        n116 = call "Init_Horizontal_ROI.vi"("error in (no error)"=w193, "input cluster"=w197) -> ("error out"=w192:errorcluster, "output cluster"=w200:T3)  [unwired: 8 in]
        n117 = disable-structure shown="Enabled" {
          disable-tunnel: w214 -> [w223 w224]
          disable-tunnel: [w222 w224] -> w213
          disable-tunnel: [w221 w225] -> w212
          disable-tunnel: "init_beamprofiler" ("function name") -> [w219 _]
          disable-tunnel: w192 -> [w216 w225]
          frame Disabled {
            n118 = local read "Beam Profiler Kwargs"() -> (w217:cluster{"Pixel Size":dbl})
            n119 = Flatten To JSON(anything=w217, error in (no error)=w216) -> (JSON string=w218:string, 11:w215:errorcluster)  [unwired: 1 in]
            n120 = node(w223, path "C:/Users/quantum/Documents/LVDAQ/Beam_Profiler_Wrapper.py" ("module path"), w219, w215, w218) -> (w222:refnum<k35>, w221:errorcluster)  [unwired: 3 in, 2 out]
          }
          frame Enabled {
          }
        }
        n121 = local read "Mode"() -> (w204:enum16{"ROI", "Image"})
        n122 = local read "Auto?"() -> (w201:bool)
        n123 = local read "Log?"() -> (w202:bool)
        n124 = Bundle By Name(cluster=w200, "Mode"=w204, "Manual LUT"=w203, "Log?"=w202, "Auto?"=w201) -> (w188:T3)
        n125 = Unbundle By Name(w188) -> ("HROI Pos"=w198:u16, "Image Type"=w191:T4, "ImageProcessed"=→"Image Processed":T2, "Image"=→"Image":T2, "ImagePreview"=→"Image Preview":T2)
        n126 = Unbundle By Name(w188) -> ("Image X"=w185:i32, "Image Y"=w184:i32)
        n127 = property on="Calibration Axes" class="IntGraph (strict)"("XScale.Maximum"=w185, "YScale.Maximum"=w184) -> (error out=w183:errorcluster)  [unwired: 2 in, 1 out]
        n128 = property on="Image Preview" class="ImageControl"(error in=w183) -> ("Displayed Image Size"=w187:cluster{"Width":u32, "Height":u32}, "Displayed Image Height"=w186:u32)  [unwired: 1 in, 2 out]
        n129 = case shown="0, Default" w191 {
          tunnel: [T6 {"Maximum"=255.0, "Minimum"=0.0, "Increment"=1.0} ("Data Entry Limits") T6 {"Maximum"=65535.0, "Minimum"=0.0, "Increment"=1.0} ("Data Entry Limits")] -> w181
          frame 0, Default {
          }
          frame 7 {
          }
        }
        n130 = property on="Manual" class="Slide (strict)"("Height"=w186) -> ()  [unwired: 2 in, 2 out]
        n131 = property on="Image Preview" class="ImageControl"("Image Area Size"=w187) -> ()  [unwired: 2 in, 2 out]
        n132 = property on="Calibration Axes" class="IntGraph (strict)"("Plot Area Size"=w187) -> ()  [unwired: 2 in, 2 out]
        n133 = property on="Manual" class="Slide (strict)"("Data Range"=w181) -> ()  [unwired: 2 in, 2 out]
        n134 = Unbundle By Name(w181) -> ("Maximum"=w178:dbl, "Minimum"=w180:dbl, "Increment"=w179:dbl)
        n135 = property on="Manual" class="Slide (strict)"("Scale.Maximum"=w178, "Scale.Minimum"=w180, "Scale.Increment"=w179) -> ()  [unwired: 2 in, 2 out]
        n136 = local write "HROI Pos"(w198) -> ()
      }
      event "Save": Value Change {
        n137 = event-data() -> ()  [unwired: 1 in, 6 out]
        n138 = Unbundle By Name(w288) -> ("ImageProcessed"=w291:T2)
        n139 = local read "File Name"() -> (w293:string)
        n140 = local read "File Path"() -> (w294:path)
        n141 = call "Save_Image.vi"("error in (no error)"=w292, "String"=w293, "Scan Save Path"=w294, "Refnum in"=w291) -> ("error out"=w290:errorcluster)  [unwired: 7 in]
      }
      event User Event {
        # "Process the image, and display the processed one"
        # "Handle Available Frames"
        n142 = event-data() -> ("Image In"=w307:T2, "Processed Frames per Second"=→"FPS":dbl)  [unwired: 1 in]
        n143 = control-ref of="ROI Graph"() -> (w308:refnum<vi>)
        n144 = call "Image_Processing.vi"("Image"=w307, "input cluster"=w306, "WaveformGraph in"=w308, "error in (no error)"=w309) -> ("output cluster"=w298:T3, "error out"=w302:errorcluster)  [unwired: 14 in]
        n145 = Unbundle By Name(w298) -> ("ROI Parameters"=w304:cluster{"Count":sgl, "Size(um)":sgl}, "Intensity Graph"=w305:u8[][], "ImagePreview"=w299:T2)
        n146 = local read "Beam Profile"() -> (w303:bool)
        n147 = case shown="False" w303 {
          tunnel: w302 -> [w317 w320]
          tunnel: [w317 w326] -> w297
          tunnel: w301 -> [w316 w330]
          tunnel: [w316 w329] -> w300
          tunnel: w299 -> [_ w321]
          frame False {
          }
          frame True {
            w325 = "calculate_values" ("function name")
            n148 = call "IMAQ ImageToArray"("error in (no error)"=w320, "Image"=w321) -> ("error out"=w318:errorcluster, "Image Pixels (U8)"=w319:u8[][])  [unwired: 2 in, 3 out]
            n149 = node(w330, path "C:/Users/quantum/Documents/LVDAQ/Beam_Profiler_Wrapper.py" ("module path"), w325, w318, w325, w319) -> (w329:refnum<k35>, w322:errorcluster, w327:string)  [unwired: 1 in, 2 out]
            n150 = Unflatten From JSON(JSON string=w327, type and defaults="Beam Profiler Data", error in (no error)=w322) -> (value=→"Beam Profile":T1, error out=w326:errorcluster)  [unwired: 4 in]
          }
        }
        n151 = local write "ROI Parameters"(w304) -> ()
        n152 = local write "Calibration Axes"(w305) -> ()
        n153 = local write "Image Processed"(w299) -> ()
        n154 = local read "Capturing"() -> (w295:bool)
        n155 = case shown="True" w295 {
          tunnel: w297 -> [w311 w313]
          tunnel: [w311 w312] -> w296
          frame False {
          }
          frame True {
            n156 = local read "Camera Enqueuer"() -> (w314:refnum<class "Message Enqueuer.lvclass">)
            n157 = local read "Image"() -> (w315:T2)
            n158 = call "Send GetFrame.vi"("error in (no error)"=w313, "Image In"=w315, "Message Enqueuer"=w314) -> ("error out"=w312:errorcluster)  [unwired: 7 in, 1 out]
          }
        }
      }
      event "Auto?", "Log?", "Manual", "Mode": Value Change {
        n159 = event-data() -> ()  [unwired: 1 in, 6 out]
        n160 = Bundle By Name(cluster=w338, "Mode"="Mode", "Manual LUT"="Manual", "Log?"="Log?", "Auto?"="Auto?") -> (w334:T3)
        n161 = control-ref of="ROI Graph"() -> (w339:refnum<vi>)
        n162 = local read "Capturing"() -> (w343:bool)
        n163 = local read "Image"() -> (w333:T2)
        n164 = case shown="False" w343 {
          tunnel: w339 -> [w351 _]
          tunnel: [w350 w353] -> w336
          tunnel: w337 -> [w349 w353]
          tunnel: w334 -> [w348 w352]
          tunnel: [w346 w352] -> w331
          tunnel: w333 -> [w347 _]
          frame False {
            n165 = call "Image_Processing.vi"("Image"=w347, "input cluster"=w348, "WaveformGraph in"=w351, "error in (no error)"=w349) -> ("output cluster"=w346:T3, "error out"=w350:errorcluster)  [unwired: 14 in]
            n166 = Unbundle By Name(w346) -> ("ImageProcessed"=w344:T2, "ROI Parameters"=→"ROI Parameters":cluster{"Count":sgl, "Size(um)":sgl})
            n167 = local write "Image Processed"(w344) -> ()
          }
          frame True {
          }
        }
      }
      event "HROI Pos": Value Change {
        n168 = event-data() -> ("NewVal"=w357:u16)  [unwired: 1 in, 5 out]
        n169 = Bundle By Name(cluster=w359, "HROI Pos"=w357) -> (w358:T3)
        n170 = local read "HROI"() -> (w356:bool)
        n171 = case shown="True" w356 {
          tunnel: w361 -> [w362 w367]
          tunnel: [w362 w366] -> w360
          tunnel: [w363 w365] -> w354
          tunnel: w358 -> [w363 w364]
          frame False {
          }
          frame True {
            n172 = call "Set_Horizontal_ROI.vi"("error in (no error)"=w367, "input cluster"=w364) -> ("error out"=w366:errorcluster, "output cluster"=w365:T3)  [unwired: 8 in]
          }
        }
      }
      event "HROI": Value Change {
        n173 = event-data() -> ("NewVal"=w372:bool)  [unwired: 1 in, 5 out]
        n174 = case shown="True" w372 {
          tunnel: w373 -> [w378 w383]
          tunnel: [w376 w382] -> w368
          tunnel: w371 -> [w375 w380]
          tunnel: [w374 w380] -> w370
          frame True {
            n175 = flat-sequence {
              tunnel: [w379] -> w377
              tunnel: w378 -> [w379]
              frame #0 {
                n176 = invoke on="Image Processed" class="ImageControl" method="Clear ROI"() -> ()  [unwired: 3 in, 3 out]
              }
            }
            n177 = call "Set_Horizontal_ROI.vi"("error in (no error)"=w375, "input cluster"=w377) -> ("error out"=w374:errorcluster, "output cluster"=w376:T3)  [unwired: 8 in]
          }
          frame False {
            n178 = Unbundle By Name(w383) -> ("Custom ROI"=w381:T7)
            n179 = Bundle By Name(cluster=w383, "ROI"=w381) -> (w382:T3)
          }
        }
      }
    }
  }
  n180 = while {
    shift-right: [w385] -> w39
    shift-left: errorcluster {"status"=FALSE, "code"=0, "source"=""} ("error out") -> [w386]
    tunnel: w45 -> [w388]
    tunnel: [w387] -> w38
    stop <- w384 stop-if-true
    n181 = event shown="[12] <Disconnected>: User Event" {
      selector: w388 -> [_ _ _ _ _ _ _ _ _ _ _ _ _ _]
      dyn-events: [_ _ _ _ _ _ _ _ _ _ _ _ _ _] -> w387
      timeout: _ -> [_ _ _ _ _ _ _ _ _ _ _ _ _ _]
      tunnel: [w390 w417 w433 w441 w450 w461 w487 w497 w503 w509 w518 w520 w526 w532] -> w385
      tunnel: w386 -> [w389 w420 w434 w442 w452 w462 w492 w497 w502 w510 w518 w521 w524 w532]
      tunnel: [_ _ _ _ _ _ _ _ _ _ _ _ _ TRUE] -> w384
      event "Open Camera": Value Change {
        n182 = event-data() -> ("NewVal"=w391:bool)  [unwired: 1 in, 5 out]
        n183 = case shown="False" w391 {
          tunnel: [w393 w397] -> w390
          tunnel: w389 -> [w394 w400]
          frame False {
            n184 = local write "Capturing"(FALSE ("Capturing")) -> ()
            n185 = local read "Camera Enqueuer"() -> (w392:refnum<class "Message Enqueuer.lvclass">)
            n186 = call "Send DeInit.vi"("error in (no error)"=w394, "Message Enqueuer"=w392) -> ("error out"=w393:errorcluster)  [unwired: 8 in, 1 out]
          }
          frame True {
            n187 = property on="Camera" class="Ring (strict)"() -> ("Value"=w407:u16)  [unwired: 2 in, 2 out]
            n188 = property on="Brand" class="Arr (strict)"() -> ("Value"=w406:string[])  [unwired: 2 in, 2 out]
            n189 = local write "Cam Enqueuer Init"(TRUE ("Initialized")) -> ()
            n190 = Index Array(array=w406, index=w407) -> (element=w405:string)
            n191 = case shown="\"INOVISION\"" w405 {
              tunnel: [refnum<class "Message Enqueuer.lvclass"> refnum ("Nested Actor's Enqueuer") w413 w416] -> w403
              tunnel: w400 -> [w408 w411 _]
              tunnel: [w408 w410 w414] -> w399
              frame "False", Default {
              }
              frame "INOVISION" {
                n192 = local read "Orca Enqueuer"() -> (w412:refnum<class "Message Enqueuer.lvclass">)
                n193 = local read "Inovance Enqueuer"() -> (w413:refnum<class "Message Enqueuer.lvclass">)
                n194 = call <vilib>:"Send Normal Stop.vi"("error in (no error)"=w411, "Message Enqueuer"=w412) -> ("error out"=w410:errorcluster)  [unwired: 9 in]
              }
              frame "Hamamatsu" {
                n195 = local read "Inovance Enqueuer"() -> (w415:refnum<class "Message Enqueuer.lvclass">)
                n196 = local read "Orca Enqueuer"() -> (w416:refnum<class "Message Enqueuer.lvclass">)
                n197 = call <vilib>:"Send Normal Stop.vi"("Message Enqueuer"=w415) -> ("error out"=w414:errorcluster)  [unwired: 10 in]
              }
            }
            "Camera Enqueuer" <- w403
            n198 = local read "Instrument Address"() -> (w402:string[])
            n199 = property on="Camera" class="Ring (strict)"() -> ("Value"=w404:u16)  [unwired: 2 in, 2 out]
            n200 = Index Array(array=w402, index=w404) -> (element=w401:string)
            n201 = call "Send Init.vi"("error in (no error)"=w400, "Address"=w401, "Message Enqueuer"=w403) -> ("error out"=w398:errorcluster)  [unwired: 7 in, 1 out]
            n202 = Merge Errors(w399, w398) -> (w397:errorcluster)
          }
        }
      }
      event "Live": Value Change {
        n203 = event-data() -> ("NewVal"=w419:bool)  [unwired: 1 in, 5 out]
        n204 = case shown="False" w419 {
          tunnel: w420 -> [w427 w431]
          tunnel: [w426 w428] -> w418
          frame True {
            n205 = local read "Camera Enqueuer"() -> (w425:refnum<class "Message Enqueuer.lvclass">)
            n206 = call "Send StartCapture.vi"("error in (no error)"=w427, "Message Enqueuer"=w425) -> ("error out"=w426:errorcluster)  [unwired: 8 in, 1 out]
          }
          frame False {
            n207 = local read "Camera Enqueuer"() -> (w429:refnum<class "Message Enqueuer.lvclass">)
            n208 = call "Send StopCapture.vi"("Message Priority (Normal)"=Message_Priority."High", "error in (no error)"=w431, "Message Enqueuer"=w429) -> ("error out"=w428:errorcluster)  [unwired: 7 in, 1 out]
          }
        }
        n209 = case shown="Error .." w418 {
          selector: w418 -> [_ w424]
          tunnel: [errorcluster {"status"=FALSE, "code"=0, "source"=""} ("error out") errorcluster {"status"=FALSE, "code"=0, "source"=""} ("error out")] -> w417
          frame No Error {
          }
          frame Error {
            n210 = Unbundle By Name(w424) -> ("source"=w423:string)
            n211 = One Button Dialog(message=w423) -> ()  [unwired: 1 in, 1 out]
          }
        }
      }
      event "Acquire": Value Change {
        n212 = event-data() -> ()  [unwired: 1 in, 6 out]
        n213 = local read "Capturing"() -> (w432:bool)
        n214 = case shown="False" w432 {
          tunnel: w434 -> [w437 w439]
          tunnel: [w436 w439] -> w433
          frame False {
            n215 = local read "Camera Enqueuer"() -> (w435:refnum<class "Message Enqueuer.lvclass">)
            n216 = local read "Image"() -> (w438:T2)
            n217 = call "Send SingleAcquisition.vi"("error in (no error)"=w437, "Image"=w438, "Message Enqueuer"=w435) -> ("error out"=w436:errorcluster)  [unwired: 7 in, 1 out]
          }
          frame True {
          }
        }
      }
      event "Exposure": Value Change {
        n218 = event-data() -> ("NewVal"=w443:dbl)  [unwired: 1 in, 5 out]
        n219 = local read "Initialized"() -> (w440:bool)
        n220 = case shown="True" w440 {
          tunnel: w443 -> [_ w449]
          tunnel: w442 -> [w444 w448]
          tunnel: [w444 w447] -> w441
          frame False {
          }
          frame True {
            n221 = local read "Camera Enqueuer"() -> (w445:refnum<class "Message Enqueuer.lvclass">)
            n222 = call "Send SetExposure.vi"("Message Priority (Normal)"=Message_Priority."High", "error in (no error)"=w448, "Exposure(ms)"=w449, "Message Enqueuer"=w445) -> ("error out"=w447:errorcluster)  [unwired: 6 in, 1 out]
          }
        }
      }
      event "Gain": Value Change {
        n223 = event-data() -> ("NewVal"=w451:dbl)  [unwired: 1 in, 5 out]
        n224 = local read "Initialized"() -> (w453:bool)
        n225 = case shown="True" w453 {
          tunnel: w451 -> [_ w459]
          tunnel: w452 -> [w454 w458]
          tunnel: [w454 w457] -> w450
          frame False {
          }
          frame True {
            n226 = local read "Camera Enqueuer"() -> (w455:refnum<class "Message Enqueuer.lvclass">)
            n227 = call "Send Set Gain.vi"("Message Priority (Normal)"=Message_Priority."High", "error in (no error)"=w458, "Gain"=w459, "Message Enqueuer"=w455) -> ("error out"=w457:errorcluster)  [unwired: 6 in, 1 out]
          }
        }
      }
      event "Stop": Value Change {
        n228 = event-data() -> ()  [unwired: 1 in, 6 out]
        n229 = local read "Cam Enqueuer Init"() -> (w460:bool)
        n230 = case shown="True" w460 {
          tunnel: w462 -> [w464 w473]
          tunnel: [w466 w471] -> w461
          frame False {
            n231 = local read "Inovance Enqueuer"() -> (w470:refnum<class "Message Enqueuer.lvclass">)
            n232 = local read "Orca Enqueuer"() -> (w465:refnum<class "Message Enqueuer.lvclass">)
            n233 = local read "Self Enqueuer"() -> (w469:refnum<class "Message Enqueuer.lvclass">)
            n234 = call <vilib>:"Send Normal Stop.vi"("error in (no error)"=w464, "Message Enqueuer"=w470) -> ("error out"=w468:errorcluster)  [unwired: 9 in]
            n235 = call <vilib>:"Send Normal Stop.vi"("error in (no error)"=w464, "Message Enqueuer"=w469) -> ("error out"=w467:errorcluster)  [unwired: 9 in]
            n236 = call <vilib>:"Send Normal Stop.vi"("error in (no error)"=w464, "Message Enqueuer"=w465) -> ("error out"=w463:errorcluster)  [unwired: 9 in]
            n237 = Merge Errors(w468, w467, w463) -> (w466:errorcluster)
          }
          frame True {
            n238 = local read "Capturing"() -> (w472:bool)
            n239 = case shown="False" w472 {
              tunnel: w473 -> [w478 w482]
              tunnel: [w474 w480] -> w471
              frame False {
                n240 = local read "Camera Enqueuer"() -> (w479:refnum<class "Message Enqueuer.lvclass">)
                n241 = call "Send DeInit.vi"("error in (no error)"=w478, "Message Enqueuer"=w479) -> ("error out"=w475:errorcluster)  [unwired: 8 in, 1 out]
                n242 = local read "Image"() -> (w477:T2)
                n243 = call "IMAQ Dispose"("All Images? (No)"=TRUE, "Image"=w477, "error in (no error)"=w475) -> ("error out"=w474:errorcluster)  [unwired: 3 in]
              }
              frame True {
                n244 = local write "Stopping"(TRUE ("Stopping")) -> ()
                n245 = local read "Camera Enqueuer"() -> (w483:refnum<class "Message Enqueuer.lvclass">)
                n246 = call "Send StopCapture.vi"("error in (no error)"=w482, "Message Enqueuer"=w483) -> ("error out"=w480:errorcluster)  [unwired: 8 in, 1 out]
              }
            }
          }
        }
      }
      event Panel Close? {
        n247 = event-data() -> ()  [unwired: 1 in, 4 out]
        n248 = local read "Initialized"() -> (w486:bool)
        n249 = case shown="True" w486 {
          tunnel: w492 -> [w493 w496]
          tunnel: [w493 w495] -> w491
          frame False {
          }
          frame True {
            n250 = local read "Camera Enqueuer"() -> (w494:refnum<class "Message Enqueuer.lvclass">)
            n251 = call "Send DeInit.vi"("error in (no error)"=w496, "Message Enqueuer"=w494) -> ("error out"=w495:errorcluster)  [unwired: 8 in, 1 out]
          }
        }
        n252 = local read "Camera Enqueuer"() -> (w485:refnum<class "Message Enqueuer.lvclass">)
        n253 = local read "Self Enqueuer"() -> (w484:refnum<class "Message Enqueuer.lvclass">)
        n254 = call <vilib>:"Send Normal Stop.vi"("error in (no error)"=w491, "Message Enqueuer"=w485) -> ()  [unwired: 9 in, 1 out]
        n255 = call <vilib>:"Send Normal Stop.vi"("error in (no error)"=w491, "Message Enqueuer"=w484) -> ("error out"=w490:errorcluster)  [unwired: 9 in]
        n256 = local read "Image"() -> (w489:T2)
        n257 = call "IMAQ Dispose"("All Images? (No)"=TRUE, "Image"=w489, "error in (no error)"=w490) -> ("error out"=w487:errorcluster)  [unwired: 3 in]
        n258 = event-data() -> ()  [unwired: 2 in, 1 out]
      }
      event User Event {
        n259 = event-data() -> ()  [unwired: 1 in, 1 out]
        n260 = local write "Initialized"(TRUE ("Initialized")) -> ()
      }
      event User Event {
        n261 = event-data() -> ()  [unwired: 1 in, 4 out]
        n262 = local read "Camera Enqueuer"() -> (w500:refnum<class "Message Enqueuer.lvclass">)
        n263 = local write "Capturing"(TRUE ("Capturing")) -> ()
        n264 = local read "Image"() -> (w499:T2)
        n265 = call "Send GetFrame.vi"("error in (no error)"=w502, "Image In"=w499, "Message Enqueuer"=w500) -> ("error out"=w501:errorcluster)  [unwired: 7 in, 1 out]
        n266 = case shown="Error .." w501 {
          selector: w501 -> [_ w508]
          tunnel: [errorcluster {"status"=FALSE, "code"=0, "source"=""} ("error out") errorcluster {"status"=FALSE, "code"=0, "source"=""} ("error out")] -> w503
          frame No Error {
          }
          frame Error {
            n267 = Unbundle By Name(w508) -> ("source"=w507:string)
            n268 = One Button Dialog(message=w507) -> ()  [unwired: 1 in, 1 out]
          }
        }
      }
      event User Event {
        n269 = event-data() -> ()  [unwired: 1 in, 4 out]
        n270 = local read "Stopping"() -> (w511:bool)
        n271 = local write "Capturing"(FALSE ("Capturing")) -> ()
        n272 = case shown="True" w511 {
          tunnel: w510 -> [w513 w515]
          tunnel: [w513 w514] -> w509
          frame False {
          }
          frame True {
            n273 = local read "Camera Enqueuer"() -> (w516:refnum<class "Message Enqueuer.lvclass">)
            n274 = call "Send DeInit.vi"("error in (no error)"=w515, "Message Enqueuer"=w516) -> ("error out"=w514:errorcluster)  [unwired: 8 in, 1 out]
          }
        }
      }
      event User Event {
        n275 = event-data() -> ("Exposure(ms)"=w517:dbl)  [unwired: 1 in, 3 out]
        n276 = local write "Exposure"(w517) -> ()
      }
      event User Event {
        n277 = event-data() -> ()  [unwired: 1 in, 4 out]
        n278 = local read "Camera Enqueuer"() -> (w519:refnum<class "Message Enqueuer.lvclass">)
        n279 = local write "Initialized"(FALSE ("Initialized")) -> ()
        n280 = call "Send Disconnect.vi"("error in (no error)"=w521, "Message Enqueuer"=w519) -> ("error out"=w520:errorcluster)  [unwired: 8 in, 1 out]
      }
      event User Event {
        n281 = event-data() -> ()  [unwired: 1 in, 5 out]
        n282 = local read "Inovance Enqueuer"() -> (w530:refnum<class "Message Enqueuer.lvclass">)
        n283 = local read "Orca Enqueuer"() -> (w525:refnum<class "Message Enqueuer.lvclass">)
        n284 = local read "Self Enqueuer"() -> (w529:refnum<class "Message Enqueuer.lvclass">)
        n285 = call <vilib>:"Send Normal Stop.vi"("error in (no error)"=w524, "Message Enqueuer"=w525) -> ("error out"=w523:errorcluster)  [unwired: 9 in]
        n286 = call <vilib>:"Send Normal Stop.vi"("error in (no error)"=w524, "Message Enqueuer"=w530) -> ("error out"=w528:errorcluster)  [unwired: 9 in]
        n287 = call <vilib>:"Send Normal Stop.vi"("error in (no error)"=w524, "Message Enqueuer"=w529) -> ("error out"=w527:errorcluster)  [unwired: 9 in]
        n288 = Merge Errors(w523, w528, w527) -> (w526:errorcluster)
      }
      event User Event {
        n289 = event-data() -> ()  [unwired: 1 in, 4 out]
      }
    }
  }
  n290 = Unregister For Events(event registration refnum=w38, error in=w39) -> ()  [unwired: 1 out]
  n291 = Close Python Session(session in=w28, error in=w30) -> (11:w29:errorcluster)
  n292 = Unregister For Events(event registration refnum=w40, error in=w29) -> ()  [unwired: 1 out]
  "Brand" <- w19
  "Instrument Address" <- w19
  "Stopping" <- FALSE ("Capturing 2")
  "Cam Enqueuer Init" <- FALSE ("Cam Enqueuer Init")
